vi "Initialise LabVIEW Text.vi"(8 "error in (no error)":errorcluster, 11 "Resource Directory":path) -> (0 "error out":errorcluster, 3 "Teapot":T1 {"Triangles"."Vertex 3"."UV"."v" min=0 max=1 step=0.1; "Triangles"."Vertex 3"."UV"."u" min=0 max=1 step=0.1; "Triangles"."Vertex 2"."UV"."v" min=0 max=1 step=0.1; "Triangles"."Vertex 2"."UV"."u" min=0 max=1 step=0.1; "Triangles"."Vertex 1"."UV"."v" min=0 max=1 step=0.1; "Triangles"."Vertex 1"."UV"."u" min=0 max=1 step=0.1})   [LabVIEW 2022 SP3, in "Application.lvlib" / "Scene.lvclass"]
uses:
  Scene.lvclass
  Scene.lvclass/Scene.ctl
  Libraries/3D/3D.lvlib
  <userlib>/_OpenG.lib/file/file.llb/Convert File Extension (Path)__ogtk.vi
  Libraries/3D/Vector 3D.ctl
  Libraries/3D/Transform.ctl
  Libraries/3D/Object.ctl
  Libraries/Raster/UV.ctl
  Libraries/Raster/Raster.lvlib
  Libraries/3D/Vertex.ctl
  Libraries/3D/Triangle.ctl
  Libraries/Raster/Rectangle Dimensions.ctl
  Libraries/Raster/Texture.ctl
  Libraries/3D/Material.ctl
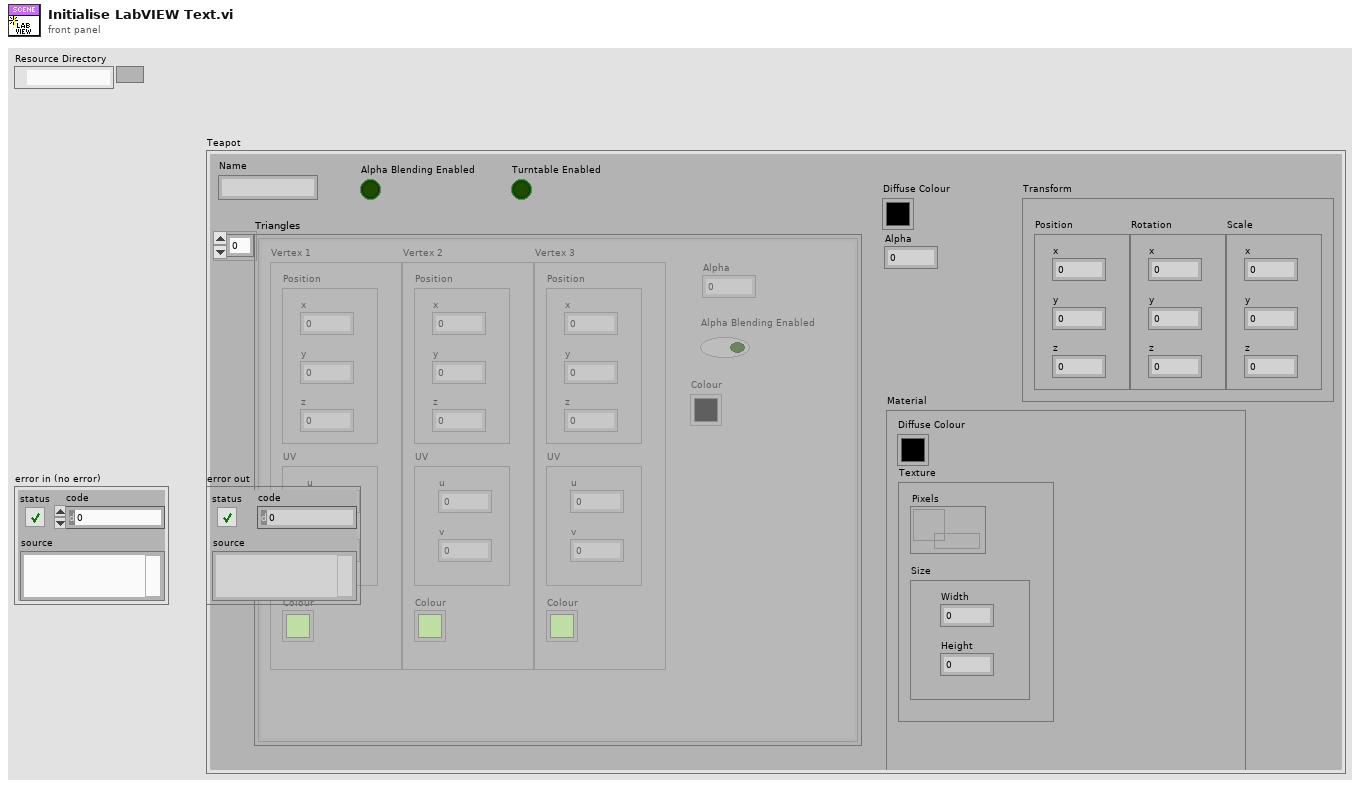
[diagram p1: front panel]
types:
  T1 = typedef "3D.lvlib/Object.ctl" = cluster{"Triangles":T2[], "Diffuse Colour":u32, "Transform":T6, "Name":string, "Alpha Blending Enabled":bool, "Alpha":dbl, "Turntable Enabled":bool, "Material":T7}
  T2 = typedef "3D.lvlib/Triangle.ctl" = cluster{"Vertex 1":T3, "Vertex 2":T3, "Vertex 3":T3, "Alpha":dbl, "Alpha Blending Enabled":bool, "Colour":u32}
  T3 = typedef "3D.lvlib/Vertex.ctl" = cluster{"Position":T4, "UV":T5, "Colour":u32}
  T4 = typedef "3D.lvlib/Vector 3D.ctl" = cluster{"x":sgl, "y":sgl, "z":sgl}
  T5 = typedef "Raster.lvlib/UV.ctl" = cluster{"u":sgl, "v":sgl}
  T6 = typedef "3D.lvlib/Transform.ctl" = cluster{"Position":T4, "Rotation":T4, "Scale":T4}
  T7 = typedef "3D.lvlib/Material.ctl" = cluster{"Diffuse Colour":u32, "Texture":T8}
  T8 = typedef "Raster.lvlib/Texture.ctl" = cluster{"Pixels":refnum<data-value>, "Size":T9}
  T9 = typedef "Raster.lvlib/Rectangle Dimensions.ctl" = cluster{"Width":u32, "Height":u32}
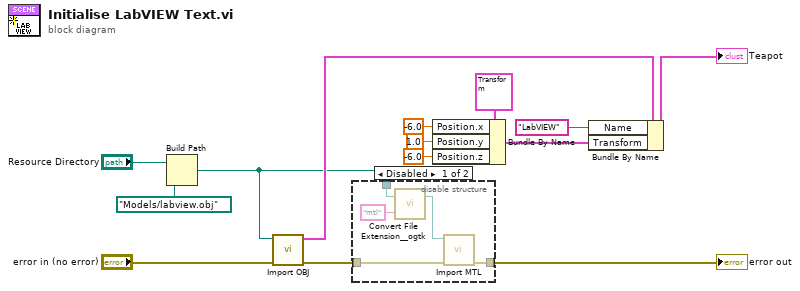
[diagram p0: block diagram]
diagram:
  n1 = Build Path(base path="Resource Directory", name or relative path=path "Models/labview.obj") -> (appended path=w1:path)
  n2 = call "Import OBJ.vi"("error in (no error)"="error in (no error)", "Object"=w1) -> ("error out"=w3:errorcluster, "Object"=w5:T1)  [unwired: 8 in]
  n3 = disable-structure shown="Disabled" {
    disable-tunnel: w3 -> [w17 _]
    disable-tunnel: [w16 _] -> w2
    disable-tunnel: w1 -> [w15 _]
    frame Disabled {
      n4 = call-poly <userlib>:"Convert File Extension__ogtk.vi"("new ending (none)"="mtl", "file name"=w15) -> ("new filename"=w19:path)  [unwired: 1 out]
      n5 = call "Import MTL.vi"("error in (no error)"=w17, "Material"=w19) -> ("error out"=w16:errorcluster)  [unwired: 8 in, 1 out]
    }
    frame Enabled {
    }
  }
  "error out" <- w2
  n6 = Bundle By Name(cluster=T6 {"Position"={"x"=2.0, "y"=1.0, "z"=-5.0}, "Rotation"={"x"=0.0, "y"=0.0, "z"=0.0}, "Scale"={"x"=0.0, "y"=0.0, "z"=0.0}} ("Transform"), "Position.x"=sgl -6.0, "Position.y"=sgl 1.0, "Position.z"=sgl -6.0) -> (w8:T6)
  n7 = Bundle By Name(cluster=w5, "Name"="LabVIEW", "Transform"=w8) -> (→"Teapot":T1)
